vi "ACDC_Config.vi"(8 "error in (no error)":errorcluster, 9 "Input Config Array":T1[](array[typedef])=[0, 0, 0, 0, 0, 0, 0, 0, 0, 0, 0, 0, 0, 0, 0, 0, 0, 0, 0, 0, 0, 0, 0, 0, 0, 0, 0, 0, 0, 0, 0, 0] items=["AC Coupled", "DC Coupled", "IEPE AC Coupled"], 10 "Data Rate [S/s]":u32) -> (0 "error out":errorcluster)   [LabVIEW 2017, in "BOP_VibAPI_4.lvlib"]
uses:
  <vilib>/addons/InsightCM/Devices/Shared/Cms/Fpga/Acquisition/source/subVIs/VibAPI_4/BOP_VibAPI_4.lvlib
  <vilib>/LabVIEW Targets/FPGA/cRIO/shared/nicrio_ModuleControls/nicrio_cRIO-9232_ConfigModeRing.ctl
  <vilib>/rvi/eio/common/nirviEmuTemplatePropertySet_errors.vi
  <vilib>/eio/EIOPropertyNode/EIOPropertyNode.xnode
  <vilib>/LabVIEW Targets/FPGA/cRIO/shared/nicrio_ModuleControls/nicrio_cRIO-9232_DataRatesRing2.ctl
  <vilib>/rvi/eio/common/nirviEmuTemplatePropertyGet_errors.vi
  <vilib>/rvi/eio/common/nirviEmuTemplatePropertyGet_noerrors.vi
  <vilib>/rvi/eio/common/nirviEmuTemplatePropertySet_noerrors.vi
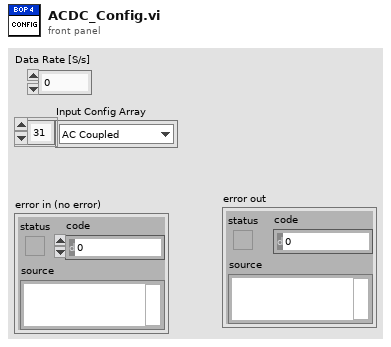
[diagram p1: front panel]
types:
  T1 = typedef "nicrio_cRIO-9232_ConfigModeRing.ctl" = u8
  T2 = typedef "nicrio_cRIO-9232_DataRatesRing2.ctl" = u8
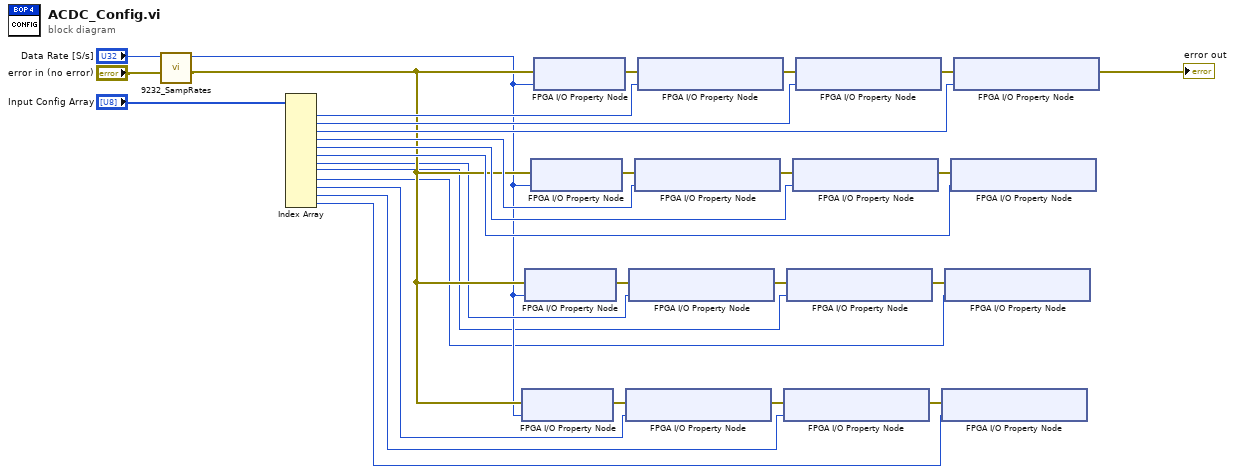
[diagram p0: block diagram]
diagram:
  n1 = call <vilib>:"9232_SampRates.vi"("error in (no error)"="error in (no error)", "Data Rate [S/s]"="Data Rate [S/s]") -> ("error out"=w8:errorcluster, "Data Rate"=w6:T2)  [unwired: 8 in]
  n2 = Index Array(array="Input Config Array") -> (element #1=w22:T1, element #2=w21:T1, element #3=w17:T1, element #4=w20:T1, element #5=w19:T1, element #6=w18:T1, element #7=w7:T1, element #8=w5:T1, element #9=w4:T1, element #10=w3:T1, element #11=w2:T1, element #12=w1:T1)  [unwired: 12 in]
  n3 = xnode "FPGA I/O Property Node"("error in"=w8, "Data Rate"=w6) -> ("error out"=w11:errorcluster)  [unwired: 1 in, 1 out]
  n4 = xnode "FPGA I/O Property Node"("error in"=w8, "Data Rate"=w6) -> ("error out"=w12:errorcluster)  [unwired: 1 in, 1 out]
  n5 = xnode "FPGA I/O Property Node"("error in"=w8, "Data Rate"=w6) -> ("error out"=w23:errorcluster)  [unwired: 1 in, 1 out]
  n6 = xnode "FPGA I/O Property Node"("error in"=w8, "Data Rate"=w6) -> ("error out"=w24:errorcluster)  [unwired: 1 in, 1 out]
  n7 = xnode "FPGA I/O Property Node"("error in"=w11, "Input Configuration"=w3) -> ("error out"=w10:errorcluster)  [unwired: 1 in, 1 out]
  n8 = xnode "FPGA I/O Property Node"("error in"=w12, "Input Configuration"=w7) -> ("error out"=w13:errorcluster)  [unwired: 1 in, 1 out]
  n9 = xnode "FPGA I/O Property Node"("error in"=w23, "Input Configuration"=w20) -> ("error out"=w27:errorcluster)  [unwired: 1 in, 1 out]
  n10 = xnode "FPGA I/O Property Node"("error in"=w24, "Input Configuration"=w22) -> ("error out"=w25:errorcluster)  [unwired: 1 in, 1 out]
  n11 = xnode "FPGA I/O Property Node"("error in"=w10, "Input Configuration"=w2) -> ("error out"=w9:errorcluster)  [unwired: 1 in, 1 out]
  n12 = xnode "FPGA I/O Property Node"("error in"=w13, "Input Configuration"=w5) -> ("error out"=w14:errorcluster)  [unwired: 1 in, 1 out]
  n13 = xnode "FPGA I/O Property Node"("error in"=w27, "Input Configuration"=w19) -> ("error out"=w28:errorcluster)  [unwired: 1 in, 1 out]
  n14 = xnode "FPGA I/O Property Node"("error in"=w25, "Input Configuration"=w21) -> ("error out"=w26:errorcluster)  [unwired: 1 in, 1 out]
  n15 = xnode "FPGA I/O Property Node"("error in"=w9, "Input Configuration"=w1) -> ()  [unwired: 1 in, 2 out]
  n16 = xnode "FPGA I/O Property Node"("error in"=w14, "Input Configuration"=w4) -> ()  [unwired: 1 in, 2 out]
  n17 = xnode "FPGA I/O Property Node"("error in"=w28, "Input Configuration"=w18) -> ()  [unwired: 1 in, 2 out]
  n18 = xnode "FPGA I/O Property Node"("error in"=w26, "Input Configuration"=w17) -> ("error out"=→"error out":errorcluster)  [unwired: 1 in, 1 out]
